vi "Start.vi"() -> ()   [LabVIEW 2025]
uses:
  <vilib>/Utility/miscctls.llb/LVPointTypeDef.ctl
  <vilib>/Utility/error.llb/Trim Whitespace One-Sided.vi
panel:
  in  "Cancel Button":bool
  in  "OK Button":bool
  in  "Software Menu":i32(ring) caption="Software Configuration" items=["Example Microscope", "OPM", "User Select"]
  in  "Hardware Menu":i32(ring) caption="Hardware Configuration" items=["Example Microscope", "OPM", "User Select"]
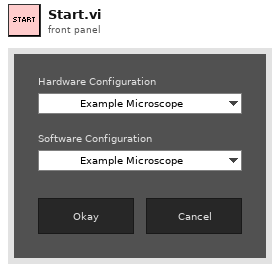
[diagram p1: front panel]
types:
  T1 = enum16{"Always On", "Always Off", "Off While Running"}
  T2 = typedef "LVPointTypeDef.ctl" = cluster{"Horizontal":i16, "Vertical":i16}
  T3 = enum32{"Invalid", "Standard", "Closed", "Hidden", "Minimized", "Maximized"}
  T4 = typedef "LVRectTypeDef.ctl" = cluster{"Left":i16, "Top":i16, "Right":i16, "Bottom":i16}
  T5 = typedef "LVBoundsTypeDef.ctl" = cluster{"Width":u32, "Height":u32}
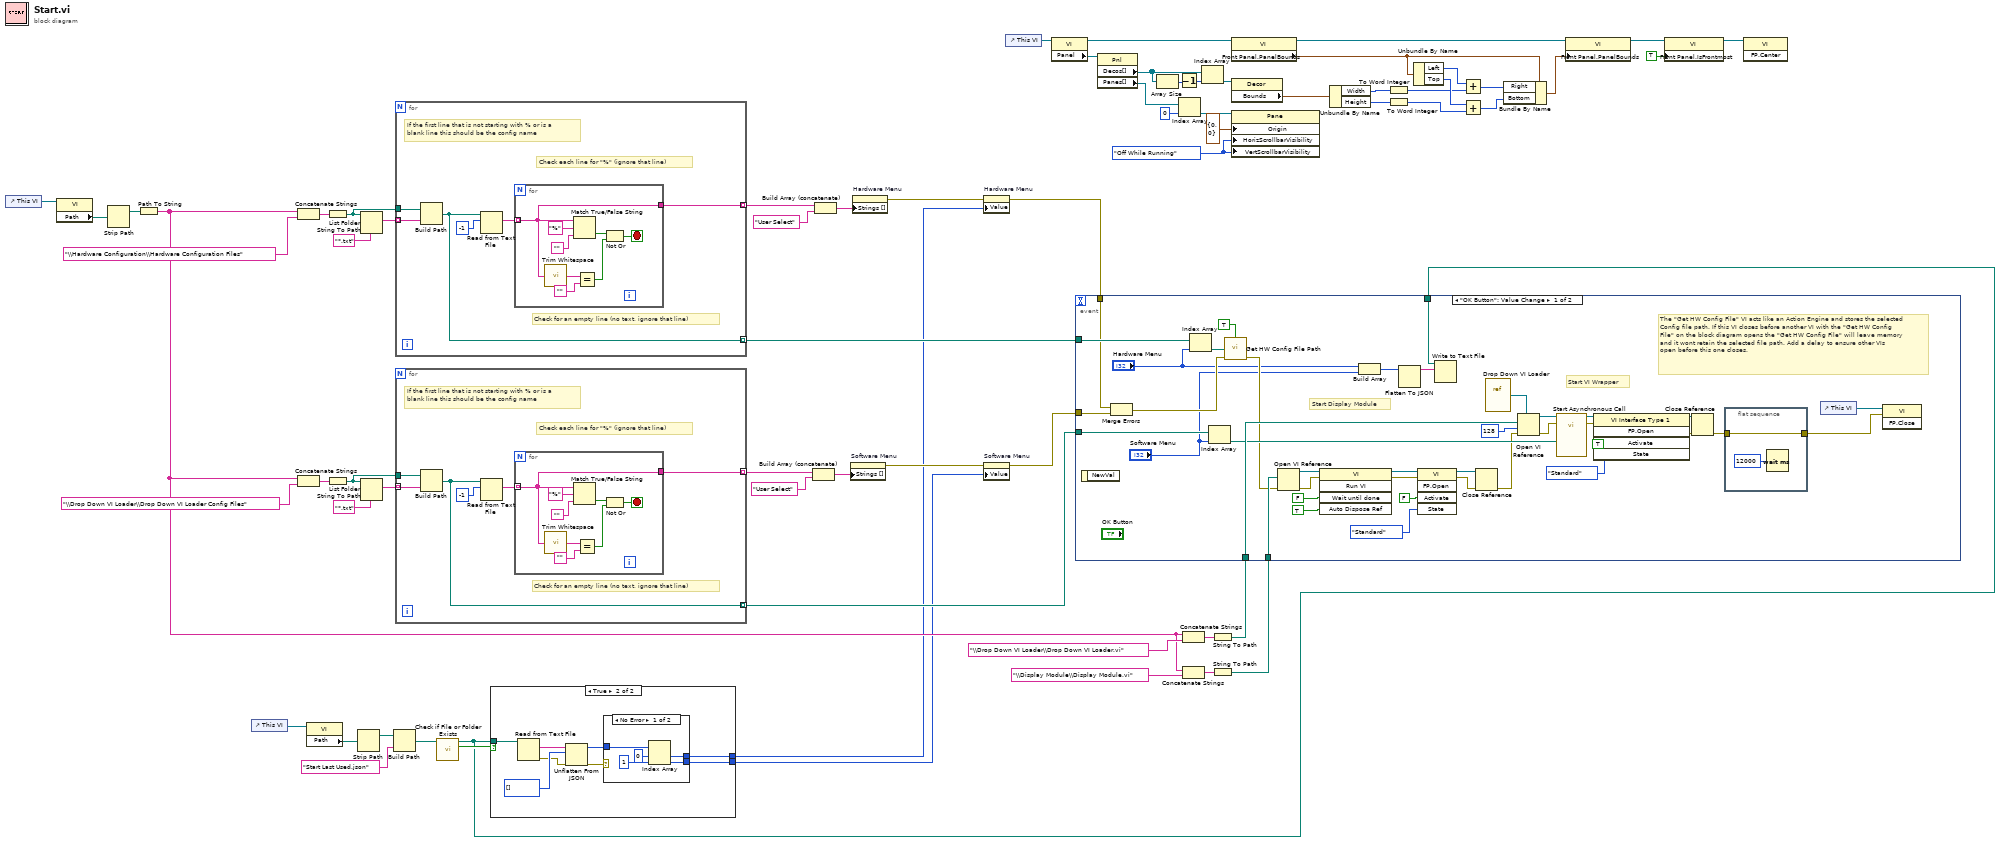
[diagram p0: block diagram]
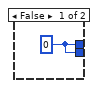
[diagram p2: hidden frame]
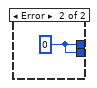
[diagram p3: hidden frame]
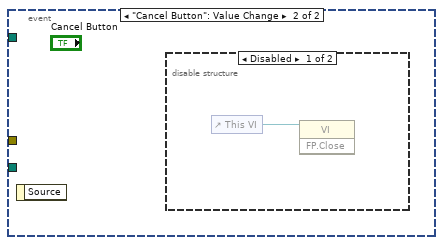
[diagram p4: hidden frame]
diagram:
  w24 = T1."Off While Running" ("Vertical Scrollbar Visibility")
  n1 = control-ref of="This VI"() -> (w68:refnum<vi>)
  n2 = property class="VI"(reference=w68) -> ("Path"=w67:path)  [unwired: 1 in, 2 out]
  n3 = Strip Path(path=w67) -> (stripped path=w66:path)  [unwired: 1 out]
  n4 = Path To String(path=w66) -> (string=w37:string)
  n5 = control-ref of="This VI"() -> (w9:refnum<vi>)
  n6 = Concatenate Strings(w37, "\\Hardware Configuration\\Hardware Configuration Files") -> (w60:string)
  n7 = Concatenate Strings(w37, "\\Drop Down VI Loader\\Drop Down VI Loader Config Files") -> (w61:string)
  n8 = property class="VI"(reference=w9) -> ("Path"=w8:path)  [unwired: 1 in, 2 out]
  n9 = String To Path(string=w60) -> (path=w58:path)
  n10 = String To Path(string=w61) -> (path=w56:path)
  n11 = Strip Path(path=w8) -> (stripped path=w7:path)  [unwired: 1 out]
  n12 = List Folder(path=w58, pattern="*.txt") -> (filenames=w59:string[])  [unwired: 2 in, 3 out]
  n13 = List Folder(path=w56, pattern="*.txt") -> (filenames=w57:string[])  [unwired: 2 in, 3 out]
  n14 = Build Path(base path=w7, name or relative path="Start Last Used.json") -> (appended path=w5:path)
  n15 = for {
    tunnel: w59 -> [w74] mode=indexing
    tunnel: w58 -> [w73]
    tunnel: [w70] -> w55 mode=indexing
    tunnel: [w69] -> w49 mode=indexing
    # "If the first line that is not starting with % or is a\nblank line this should be the config name"
    # "Check for an empty line (no text, ignore that line)"
    # "Check each line for \"%\" (ignore that line)"
    n16 = Build Path(base path=w73, name or relative path=w74) -> (appended path=w69:path)
    n17 = Read from Text File(file (use dialog)=w69, count=-1) -> (text=w72:string[])  [unwired: 2 in, 3 out]
    n18 = for {
      tunnel: w72 -> [w75] mode=indexing
      tunnel: [w75] -> w70
      stop <- w76 stop-if-true
      n19 = call <vilib>:"Trim Whitespace.vi"("string"=w75) -> ("trimmed string"=w80:string)  [unwired: 1 in]
      n20 = Match True/False String(2:"", 3:"%" ("true string"), 4:w75) -> (0:w78:bool)  [unwired: 1 out]
      n21 = Equal?(x=w80, y="") -> (x = y?=w77:bool)
      n22 = Not Or(1:w77, 2:w78) -> (0:w76:bool)
    }
  }
  n23 = for {
    tunnel: w57 -> [w88] mode=indexing
    tunnel: w56 -> [w87]
    tunnel: [w84] -> w53 mode=indexing
    tunnel: [w83] -> w48 mode=indexing
    # "If the first line that is not starting with % or is a\nblank line this should be the config name"
    # "Check for an empty line (no text, ignore that line)"
    # "Check each line for \"%\" (ignore that line)"
    n24 = Build Path(base path=w87, name or relative path=w88) -> (appended path=w83:path)
    n25 = Read from Text File(file (use dialog)=w83, count=-1) -> (text=w86:string[])  [unwired: 2 in, 3 out]
    n26 = for {
      tunnel: w86 -> [w89] mode=indexing
      tunnel: [w89] -> w84
      stop <- w90 stop-if-true
      n27 = call <vilib>:"Trim Whitespace.vi"("string"=w89) -> ("trimmed string"=w94:string)  [unwired: 1 in]
      n28 = Match True/False String(2:"", 3:"%" ("true string"), 4:w89) -> (0:w92:bool)  [unwired: 1 out]
      n29 = Equal?(x=w94, y="") -> (x = y?=w91:bool)
      n30 = Not Or(1:w91, 2:w92) -> (0:w90:bool)
    }
  }
  n31 = call <vilib>:"Check if File or Folder Exists.vi"("path"=w5) -> ("file or folder exists?"=w4:bool, "dup path"=w1:path)  [unwired: 8 in, 1 out]
  n32 = case shown="True" w4 {
    tunnel: w1 -> [_ w105]
    tunnel: [w97 w99] -> w3
    tunnel: [w97 w98] -> w2
    frame False {
      w97 = 0
    }
    frame True {
      n33 = Read from Text File(file (use dialog)=w105) -> (text=w104:string, error out=w102:errorcluster)  [unwired: 3 in, 2 out]
      n34 = Unflatten From JSON(JSON string=w104, type and defaults=i32[] [], error in (no error)=w102) -> (value=w100:i32[], error out=w101:errorcluster)  [unwired: 4 in]
      n35 = case shown="No Error" w101 {
        tunnel: w100 -> [w110 _]
        tunnel: [w107 w111] -> w99
        tunnel: [w106 w111] -> w98
        frame No Error {
          n36 = Index Array(array=w110, index #1=0 ("index"), index #2=1 ("index")) -> (element #1=w107:i32, element #2=w106:i32)
        }
        frame Error {
          w111 = 0
        }
      }
    }
  }
  n37 = Build Array (concatenate)(w53, "User Select" ("string")) -> (w51:string[])
  n38 = Build Array (concatenate)(w55, "User Select" ("string")) -> (w50:string[])
  n39 = property on="Software Menu" class="Ring (strict)"("Strings []"=w51) -> (error out=w47:errorcluster)  [unwired: 2 in, 1 out]
  n40 = property on="Hardware Menu" class="Ring (strict)"("Strings []"=w50) -> (error out=w45:errorcluster)  [unwired: 2 in, 1 out]
  n41 = property on="Hardware Menu" class="Ring (strict)"(error in=w45, "Value"=w3) -> (error out=w44:errorcluster)  [unwired: 1 in, 1 out]
  n42 = property on="Software Menu" class="Ring (strict)"(error in=w47, "Value"=w2) -> (error out=w46:errorcluster)  [unwired: 1 in, 1 out]
  n43 = control-ref of="This VI"() -> (w17:refnum<vi>)
  n44 = property class="VI"(reference=w17) -> (reference out=w25:refnum<vi>, "Panel"=w18:refnum<vi>)  [unwired: 1 in, 1 out]
  n45 = property class="Pnl"(reference=w18) -> ("Decos[]"=w16:refnum<vi>[], "Panes[]"=w21:refnum<vi>[])  [unwired: 1 in, 2 out]
  n46 = Array Size(array=w16) -> (size(s)=w14:i32)
  n47 = Decrement(x=w14) -> (x-1=w15:i32)
  n48 = Index Array(array=w21, index=0) -> (element=w20:refnum<vi>)
  n49 = Concatenate Strings(w37, "\\Drop Down VI Loader\\Drop Down VI Loader.vi") -> (w42:string)
  n50 = Concatenate Strings(w37, "\\Display Module\\Display Module.vi") -> (w40:string)
  n51 = Index Array(array=w16, index=w15) -> (element=w23:refnum<vi>)
  n52 = String To Path(string=w42) -> (path=w41:path)
  n53 = String To Path(string=w40) -> (path=w38:path)
  n54 = event shown="[0] \"OK Button\": Value Change" {
    selector: _ -> [_ _]
    dyn-events: _ -> [_ _]
    timeout: _ -> [_ _]
    tunnel: w49 -> [w151 _]
    tunnel: w48 -> [w150 _]
    tunnel: w46 -> [w143 _]
    tunnel: w44 -> [w144 _]
    tunnel: w41 -> [w149 _]
    tunnel: w38 -> [w147 _]
    tunnel: w1 -> [w112 _]
    event "OK Button": Value Change {
      # "The \"Get HW Config File\" VI acts like an Action Engine and stores the selected Config file path. If this VI closes before another VI with the \"Get HW Config File\" on the block diagram opens the \"Get HW Config File\" will leave memory and it wont retain the selected file path. Add a delay to ensure other VIs open before this one closes."
      # "Start VI Wrapper"
      # "Start Display Module"
      n55 = event-data() -> ()  [unwired: 1 in, 1 out]
      n56 = Merge Errors(w144, w143) -> (w142:errorcluster)
      n57 = Index Array(array=w151, index="Hardware Menu") -> (element=w146:path)
      n58 = Index Array(array=w150, index="Software Menu") -> (element=w148:path)
      n59 = call "Get HW Config File Path.vi"("Reset/Set File Path (F)?"=TRUE, "File Path"=w146, "Error"=w142) -> ("Error"=w120:errorcluster)  [unwired: 11 in, 1 out]
      n60 = Open VI Reference(vi path=w147, error in (no error)=w120) -> (vi reference=w134:refnum<vi>, error out=w121:errorcluster)  [unwired: 4 in]
      n61 = invoke class="VI" method="Run VI"(reference=w134, error in=w121, "Wait until done"=FALSE ("Wait Until Done"), "Auto Dispose Ref"=TRUE ("Auto Dispose Reference")) -> (reference out=w131:refnum<vi>, error out=w122:errorcluster)  [unwired: 1 in, 3 out]
      n62 = Build Array("Hardware Menu", "Software Menu") -> (w114:i32[])
      n63 = Flatten To JSON(anything=w114) -> (JSON string=w113:string)  [unwired: 2 in, 1 out]
      n64 = invoke class="VI" method="FP.Open"(reference=w131, error in=w122, "Activate"=FALSE ("Activate?"), "State"=T3."Standard") -> (reference out=w128:refnum<vi>, error out=w123:errorcluster)  [unwired: 1 in, 3 out]
      n65 = Write to Text File(file (use dialog)=w112, text=w113) -> ()  [unwired: 2 in, 3 out]
      n66 = Close Reference(reference=w128, error in (no error)=w123) -> (error out=w124:errorcluster)
      n67 = vi-ref "Drop Down VI Loader.vi"() -> (w140:refnum<vi>)
      n68 = Open VI Reference(type specifier VI Refnum (for type only)=w140, vi path=w149, options=128, error in (no error)=w124) -> (vi reference=w139:refnum<vi>, error out=w127:errorcluster)  [unwired: 2 in]
      n69 = call-by-ref "Start Asynchronous Call"(reference=w139, error in=w127, "Software Config File Path"=w148) -> (reference out=w138:refnum<vi>, error out=w126:errorcluster)  [unwired: 15 in]
      n70 = invoke class="VI Interface Type 1" method="FP.Open"(reference=w138, error in=w126, "Activate"=TRUE ("Activate?"), "State"=T3."Standard") -> (reference out=w135:refnum<vi>, error out=w125:errorcluster)  [unwired: 1 in, 3 out]
      n71 = Close Reference(reference=w135, error in (no error)=w125) -> (error out=w119:errorcluster)
      n72 = flat-sequence {
        tunnel: w119 -> [w152]
        tunnel: [w152] -> w117
        frame #0 {
          n73 = Wait (ms)(milliseconds to wait=u32 12000) -> ()  [unwired: 1 out]
        }
      }
      n74 = control-ref of="This VI"() -> (w118:refnum<vi>)
      n75 = invoke class="VI" method="FP.Close"(reference=w118, error in=w117) -> ()  [unwired: 1 in, 3 out]
    }
    event "Cancel Button": Value Change {
      n76 = event-data() -> ()  [unwired: 1 in, 1 out]
      n77 = disable-structure shown="Disabled" {
        frame Disabled {
          n78 = control-ref of="This VI"() -> (w154:refnum<vi>)
          n79 = invoke class="VI" method="FP.Close"(reference=w154) -> ()  [unwired: 2 in, 3 out]
        }
        frame Enabled {
        }
      }
    }
  }
  n80 = property class="VI"(reference=w25) -> (reference out=w27:refnum<vi>, "Front Panel.PanelBounds"=w28:T4)  [unwired: 1 in, 1 out]
  n81 = property class="Decor"(reference=w23) -> ("Bounds"=w26:T5)  [unwired: 1 in, 2 out]
  n82 = property class="Pane"(reference=w20, "Origin"=T2 {"Horizontal"=0, "Vertical"=0}, "HorizScrollbarVisibility"=w24, "VertScrollbarVisibility"=w24) -> ()  [unwired: 1 in, 2 out]
  n83 = Unbundle By Name(w26) -> ("Width"=w31:u32, "Height"=w34:u32)
  n84 = To Word Integer(number=w31) -> (16bit integer=w33:i16)
  n85 = To Word Integer(number=w34) -> (16bit integer=w13:i16)
  n86 = Unbundle By Name(w28) -> ("Left"=w30:i16, "Top"=w36:i16)
  n87 = Add(x=w30, y=w33) -> (x+y=w32:i16)
  n88 = Add(x=w36, y=w13) -> (x+y=w35:i16)
  n89 = Bundle By Name(cluster=w28, "Right"=w32, "Bottom"=w35) -> (w29:T4)
  n90 = property class="VI"(reference=w27, "Front Panel.PanelBounds"=w29) -> (reference out=w12:refnum<vi>)  [unwired: 1 in, 1 out]
  n91 = property class="VI"(reference=w12, "Front Panel.IsFrontmost"=TRUE ("Front Panel Window:Is Frontmost")) -> (reference out=w10:refnum<vi>)  [unwired: 1 in, 1 out]
  n92 = invoke class="VI" method="FP.Center"(reference=w10) -> ()  [unwired: 2 in, 3 out]
